vi "Add Result.vi"(8 "error in (no error)":errorcluster, 10 "Test Result.lvclass":refnum<class "Test Result.lvclass">, 11 "Results Manager in":refnum<class "Results Manager.lvclass">) -> (0 "error out":errorcluster, 3 "Results Manager out":refnum<class "Results Manager.lvclass">)   [LabVIEW 2021, in "Sequence Engine.lvlib" / "Results Manager.lvclass"]
uses:
  Results Manager.lvclass
  Test Result/Test Result.lvclass
  Results Manager.lvclass/Results Manager.ctl
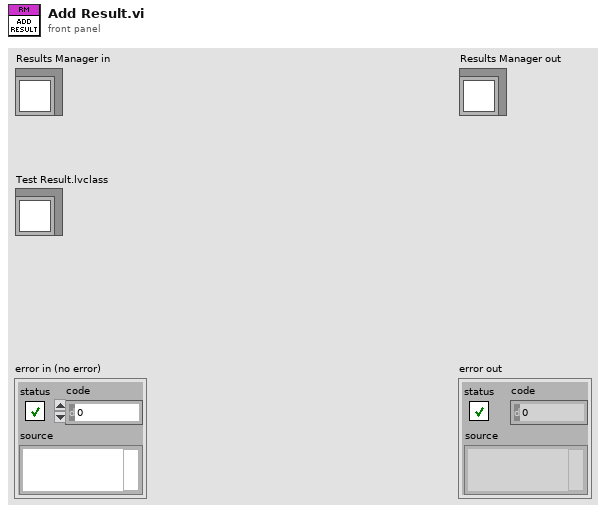
[diagram p1: front panel]
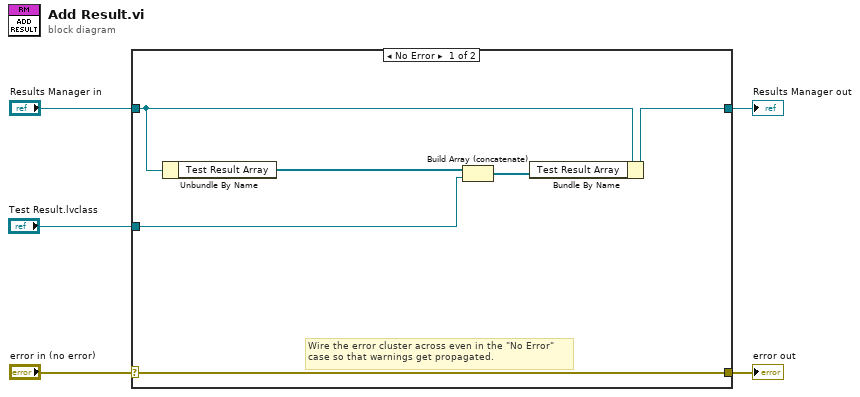
[diagram p0: block diagram]
diagram:
  n1 = case shown="No Error" "error in (no error)" {
    selector: "error in (no error)" -> [w11 w13]
    tunnel: [w11 w13] -> w4
    tunnel: [w10 w12] -> w2
    tunnel: "Results Manager in" -> [w9 w12]
    tunnel: "Test Result.lvclass" -> [w6 _]
    frame No Error {
      # "Wire the error cluster across even in the \"No Error\"\ncase so that warnings get propagated."
      n2 = Unbundle By Name(w9) -> ("Test Result Array"=w8:refnum<class "Test Result.lvclass">[])
      n3 = Build Array (concatenate)(w8, w6) -> (w7:refnum<class "Test Result.lvclass">[])
      n4 = Bundle By Name(cluster=w9, "Test Result Array"=w7) -> (w10:refnum<class "Results Manager.lvclass">)
    }
    frame Error {
    }
  }
  "error out" <- w4
  "Results Manager out" <- w2
